vi "ProcessRegistry.vi"(8 "error in (no error)":errorcluster, 11 "pSubSystem in":refnum<class "JKI SMO.lvclass">) -> (0 "error out":errorcluster, 3 "pSubSystem out":refnum<class "JKI SMO.lvclass">)   [LabVIEW 2013, in "JKI SMO.lvclass"]
doc: "This is the process registry.\n\nNote: This method must be overridden by descendant\n\n---------------------------------------------------------------\nCopyright © 2014 JKI All rights reserved.\nAuthor: Philippe Guerit <philippe.guerit@jki.net>\nThis library is provided \"AS IS\" , WITHOUT WARRANTIES OR \nCONDITIONS OF ANY KIND, either express or implied.\nJKI. -- jki.net"
uses:
  JKI SMO.lvclass
panel:
  # "Copyright © 2014 JKI All rights reserved.\n\nAuthor: Philippe Guerit <philippe.guerit@jki.net>\n\nThis library is provided \"AS IS\" , WITHOUT WARRANTIES OR \nCONDITIONS OF ANY KIND, either express or implied.\n\nJKI. -- jki.net"
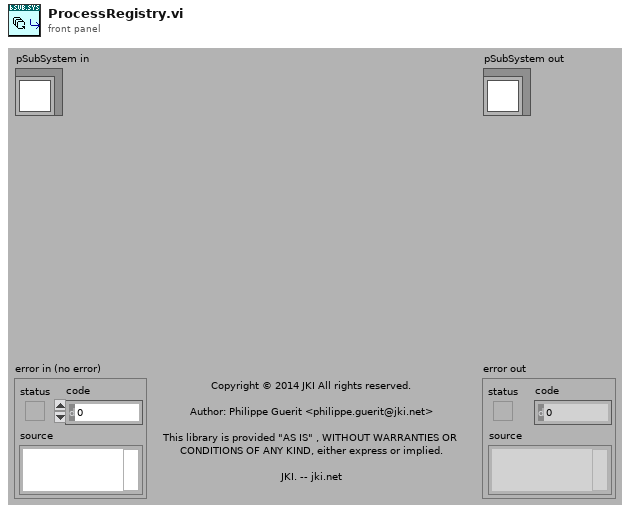
[diagram p1: front panel]
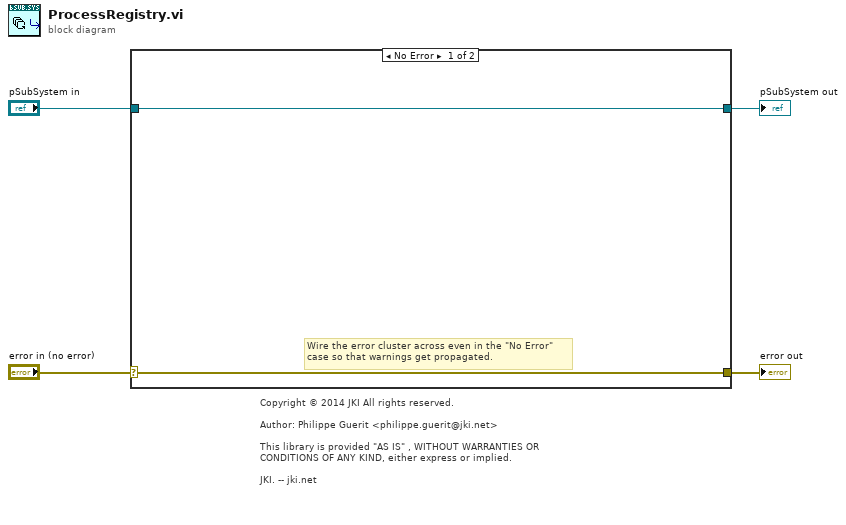
[diagram p0: block diagram]
diagram:
  # "Copyright © 2014 JKI All rights reserved.\n\nAuthor: Philippe Guerit <philippe.guerit@jki.net>\n\nThis library is provided \"AS IS\" , WITHOUT WARRANTIES OR \nCONDITIONS OF ANY KIND, either express or implied.\n\nJKI. -- jki.net"
  n1 = case shown="No Error" "error in (no error)" {
    selector: "error in (no error)" -> [w5 w8]
    tunnel: [w5 w8] -> w3
    tunnel: [w6 w7] -> w1
    tunnel: "pSubSystem in" -> [w6 w7]
    frame No Error {
      # "Wire the error cluster across even in the \"No Error\"\ncase so that warnings get propagated."
    }
    frame Error {
    }
  }
  "error out" <- w3
  "pSubSystem out" <- w1
